vi "LoadCCDmode.vi"(8 "error in (no error)":errorcluster, 11 "S4GUI in":refnum<class "S4GUI.lvclass">) -> (0 "error out":errorcluster, 3 "S4GUI out":refnum<class "S4GUI.lvclass">)   [LabVIEW 2018, in "S4GUI.lvclass"]
uses:
  S4GUI.lvclass
  S4GUI.lvclass/S4GUI.ctl
  Acquisition/Acquisition.lvclass
  Interface/Interface.lvclass
  Channel/Channel.lvclass
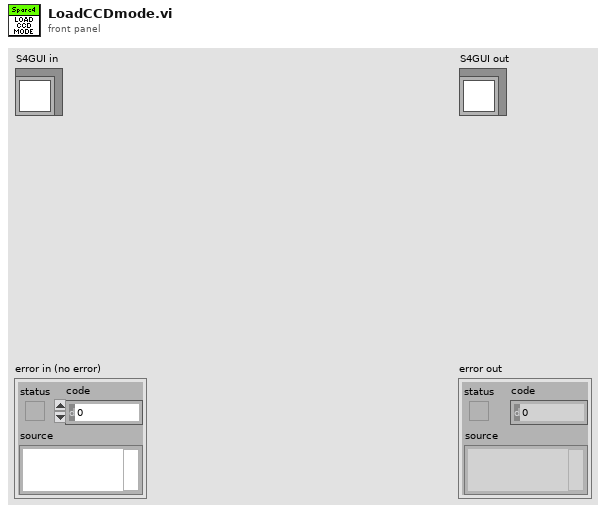
[diagram p1: front panel]
types:
  T1 = enum16{"SLOW BRIGHT: Conventional; 0.1 MHz; Gain 1", "SLOW FAINT: Conventional; 0.1 MHz; Gain 2", "NORMAL BRIGHT: Conventional; 1 MHz; Gain 1", "NORMAL FAINT: Conventional; 1 MHz; Gain 2", "FAST: EM; 10 MHz", "FAST+: EM; 20 MHz", "SUPERFAST: EM; 30 MHz"}
  T2 = enum16{"LARGE: FoV=5.6' / Pix=0.3\"", "LARGE: FoV=5.6' / Pix=0.7\"", "MEDIUM: FoV=2.8'/ Pix=0.3\"", "MEDIUM: FoV=2.8' / Pix=0.7\"", "SMALL FoV=1.4' / Pix=0.3\"", "SMALL: FoV=1.4' / Pix=0.7\""}
  T3 = cluster{"AcqRate":dbl, "MinExpTime":dbl, "readNoise":dbl, "readTime":dbl, "SatLim":dbl}
  T4 = cluster{"Image \nInitial Line":u16, "Image\nInitial Column":u16, "Image\nFinal Line":u16, "Image\nFInal Column":u16, "Vertical\nBinning":u16, "Horizontal\nBinning":u16, "Pre-amplification\nGain":u8, "CCD\nEM Gain":u16, "Readout\nRate":u8, "Shutter\nOpenning Time":i32, "Shutter\nClosing Time":i32, "Vertical\nShift Speed":u8, "Read\nMode":u8, "Vertical\nClock Voltage":u8, "A/D \nChannel":u32, "Shutter\nMode":u16, "Shutter\nTTL":u16, "Trigger\nMode":u16, "Frame\nTransfer":bool, "Acquisition\nMode":u8, "CCD \nEM Mode":u8}
  T5 = cluster{"ACQUISITION_MODE":u8, "TRIGGER_MODE":u8, "READ_MODE":u8, "PREAMP":u8, "READOUT_RATE":u8, "VERTICAL_SHIFT_SPEED":u8, "EM_MODE":u8, "EM_GAIN":u16, "SHUTTER_MODE":u8, "SHUTTER_TTL":u8, "SHUTTER_OPENING_TIME":u16, "SHUTTER_CLOSING_TIME":u16, "VBIN":u16, "HBIN":u16, "INITIAL_LINE":u16, "INITIAL_COLUMN":u16, "FINAL_LINE":u16, "FINAL_COLUMN":u16, "FRAME_TRANSFER":bool, "VERTICAL_CLOCK_VOLTAGE":u8, "AD_CHANNEL":u32}
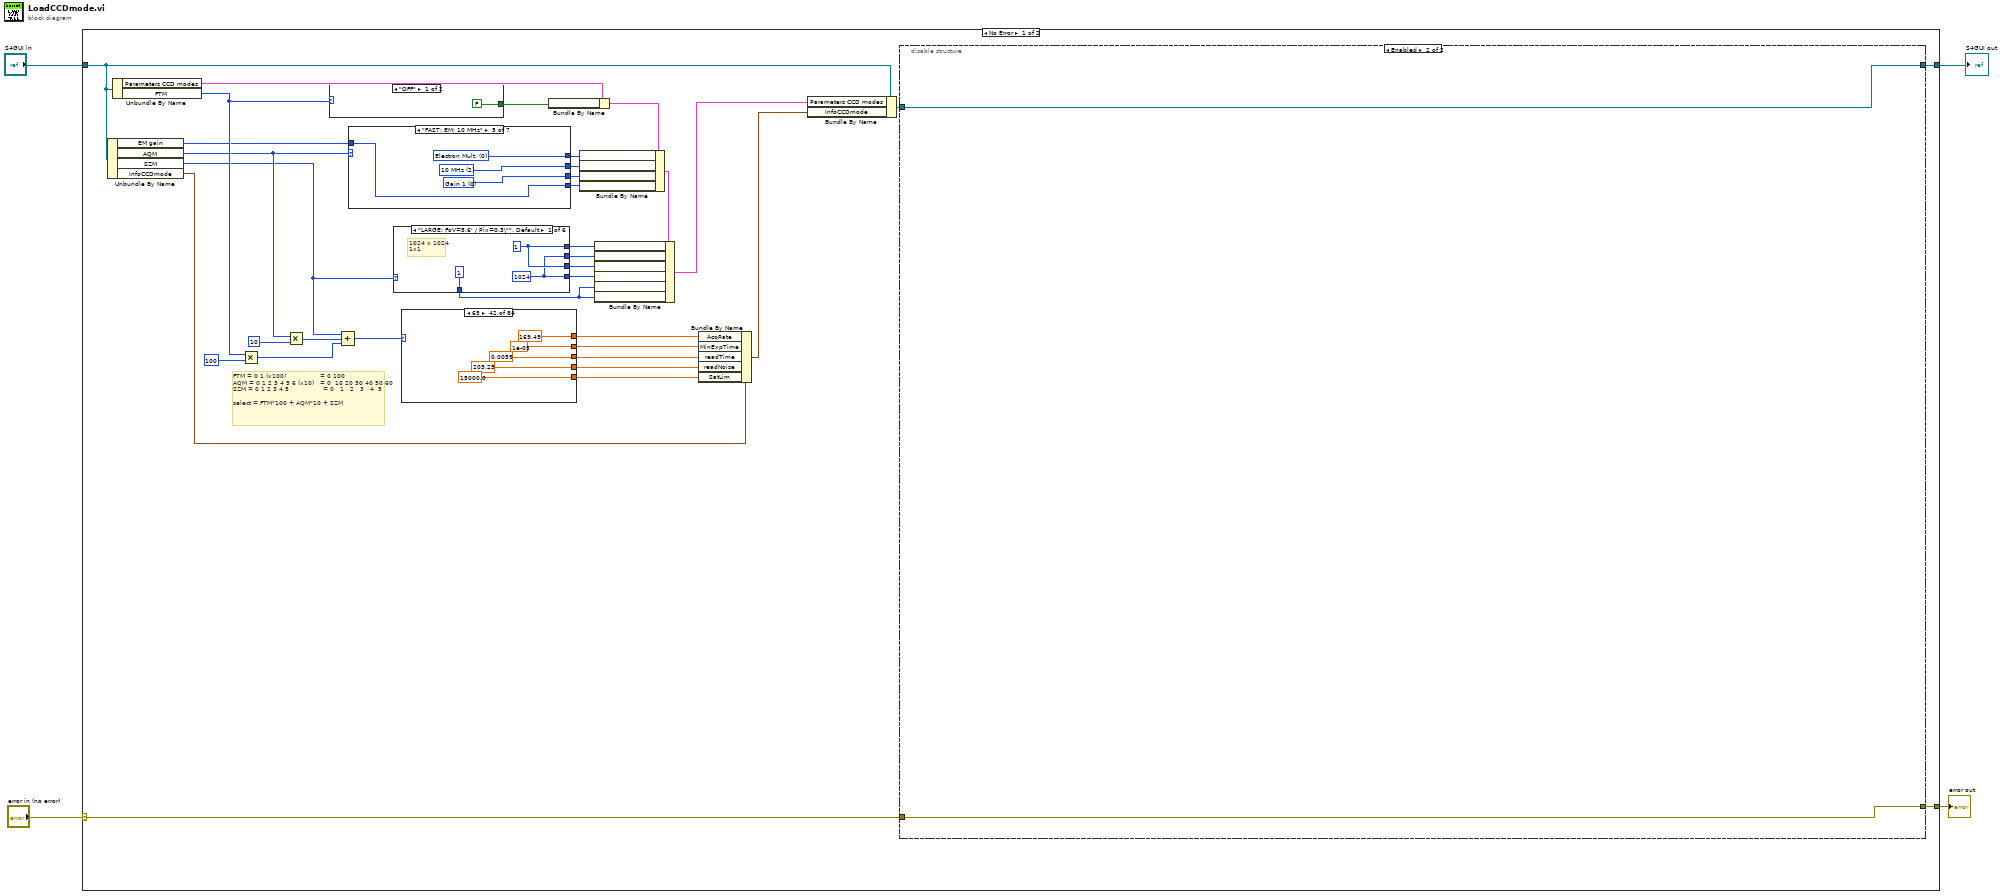
[diagram p0: block diagram]
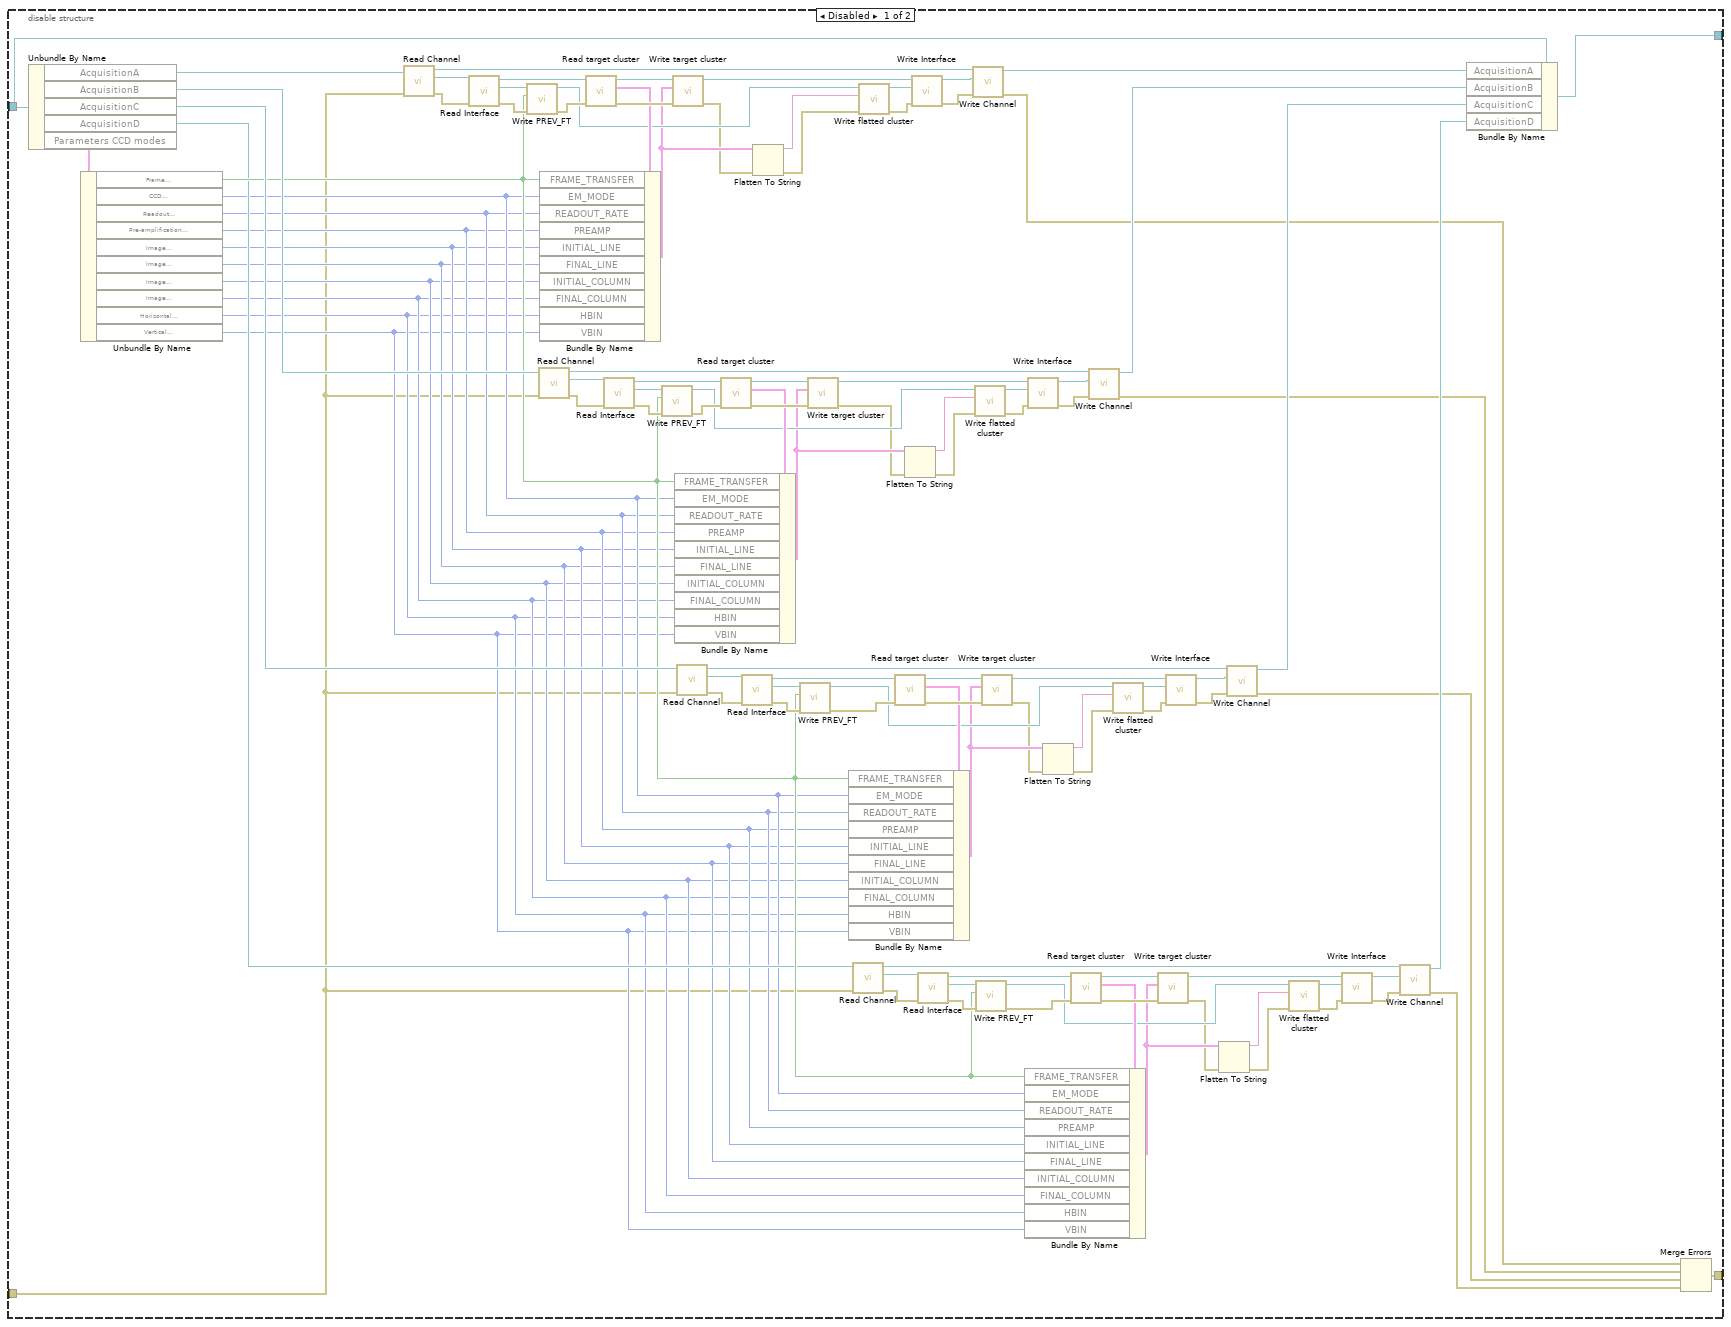
[diagram p2: hidden frame]
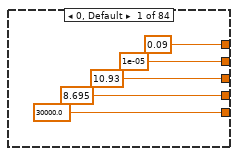
[diagram p3: hidden frame]
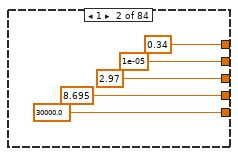
[diagram p4: hidden frame]
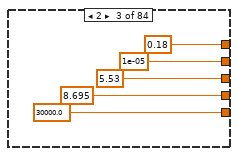
[diagram p5: hidden frame]
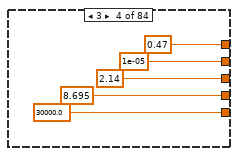
[diagram p6: hidden frame]
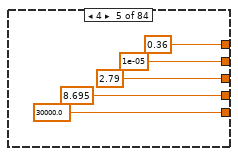
[diagram p7: hidden frame]
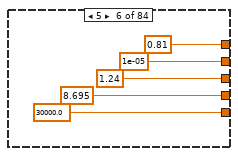
[diagram p8: hidden frame]
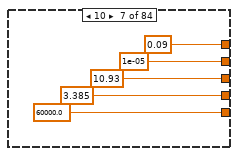
[diagram p9: hidden frame]
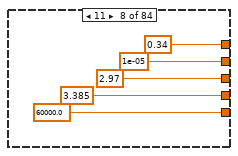
[diagram p10: hidden frame]
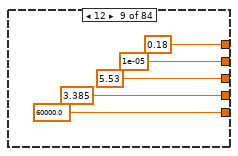
[diagram p11: hidden frame]
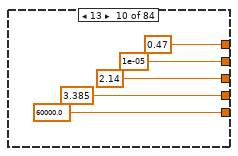
[diagram p12: hidden frame]
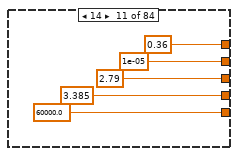
[diagram p13: hidden frame]
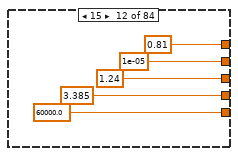
[diagram p14: hidden frame]
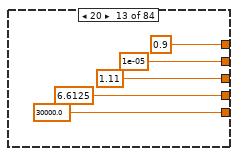
[diagram p15: hidden frame]
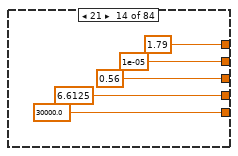
[diagram p16: hidden frame]
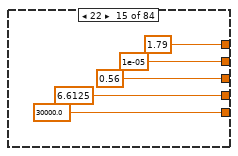
[diagram p17: hidden frame]
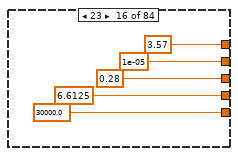
[diagram p18: hidden frame]
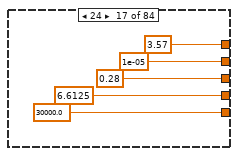
[diagram p19: hidden frame]
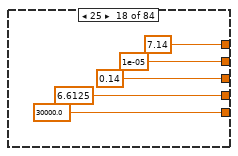
[diagram p20: hidden frame]
diagram:
  n1 = case shown="No Error" "error in (no error)" {
    selector: "error in (no error)" -> [w25 w618]
    tunnel: [w24 w618] -> w3
    tunnel: [w27 w617] -> w1
    tunnel: "S4GUI in" -> [w26 w617]
    frame No Error {
      # "FTM = 0 1 (x100)                 = 0 100\nAQM = 0 1 2 3 4 5 6 (x10)   = 0  10 20 30 40 50 60\nSZM = 0 1 2 3 4 5                 = 0   1   2   3   4  5\n\nselect = FTM*100 + AQM*10 + SZM"
      n2 = Unbundle By Name(w26) -> ("EM gain"=w5:u16, "AQM"=w8:T1, "SZM"=w7:T2, "InfoCCDmode"=w22:T3)
      n3 = Unbundle By Name(w26) -> ("Parameters CCD modes"=w20:T4, "FTM"=w9:enum16{"OFF", "ON"})
      n4 = Multiply(x=w9, y=100) -> (x*y=w11:i32)
      n5 = Multiply(x=w8, y=10) -> (x*y=w14:i32)
      n6 = case shown="\"OFF\"" w9 {
        tunnel: [FALSE TRUE] -> w39
        frame "OFF" {
        }
        frame "ON", Default {
        }
      }
      n7 = Compound Arithmetic op=ADD(w7, w14, w11) -> (w10:i32)
      n8 = case shown="\"FAST: EM; 10 MHz\"" w8 {
        tunnel: [w590 w594 w598 w602 w606 w610 w614] -> w37
        tunnel: [w589 w593 w597 w601 w604 w608 w612] -> w36
        tunnel: [w588 w592 w596 w600 w605 w609 w613] -> w35
        tunnel: [u16 2 u16 2 u16 2 u16 2 w603 w607 w611] -> w6
        tunnel: w5 -> [_ _ _ _ w603 w607 w611]
        frame "SLOW BRIGHT: Conventional; 0.1 MHz; Gain 1" {
          w588 = u8 0 items=["Gain 1", "Gain 2"] ("Pre-amplification\nGain")
          w589 = u8 1 items=["1 MHz", "0.1 MHz"] ("Readout\nRate")
          w590 = u8 1 items=["Electron Mult.", "Conventional"] ("CCD \nEM Mode")
        }
        frame "SLOW FAINT: Conventional; 0.1 MHz; Gain 2" {
          w592 = u8 1 items=["Gain 1", "Gain 2"] ("Pre-amplification\nGain")
          w593 = u8 1 items=["1 MHz", "0.1 MHz"] ("Readout\nRate")
          w594 = u8 1 items=["Electron Mult.", "Conventional"] ("CCD \nEM Mode")
        }
        frame "NORMAL BRIGHT: Conventional; 1 MHz; Gain 1", Default {
          w596 = u8 0 items=["Gain 1", "Gain 2"] ("Pre-amplification\nGain")
          w597 = u8 0 items=["1 MHz", "0.1 MHz"] ("Readout\nRate")
          w598 = u8 1 items=["Electron Mult.", "Conventional"] ("CCD \nEM Mode")
        }
        frame "NORMAL FAINT: Conventional; 1 MHz; Gain 2" {
          w600 = u8 1 items=["Gain 1", "Gain 2"] ("Pre-amplification\nGain")
          w601 = u8 0 items=["1 MHz", "0.1 MHz"] ("Readout\nRate")
          w602 = u8 1 items=["Electron Mult.", "Conventional"] ("CCD \nEM Mode")
        }
        frame "FAST: EM; 10 MHz" {
          w604 = u8 2 items=["30 MHz", "20 MHz", "10 MHz"] ("Readout\nRate")
          w605 = u8 0 items=["Gain 1", "Gain 2"] ("Pre-amplification\nGain")
          w606 = u8 0 items=["Electron Mult.", "Conventional"] ("CCD \nEM Mode")
        }
        frame "FAST+: EM; 20 MHz" {
          w608 = u8 1 items=["30 MHz", "20 MHz", "10 MHz"] ("Readout\nRate")
          w609 = u8 0 items=["Gain 1", "Gain 2"] ("Pre-amplification\nGain")
          w610 = u8 0 items=["Electron Mult.", "Conventional"] ("CCD \nEM Mode")
        }
        frame "SUPERFAST: EM; 30 MHz" {
          w612 = u8 0 items=["30 MHz", "20 MHz", "10 MHz"] ("Readout\nRate")
          w613 = u8 0 items=["Gain 1", "Gain 2"] ("Pre-amplification\nGain")
          w614 = u8 0 items=["Electron Mult.", "Conventional"] ("CCD \nEM Mode")
        }
      }
      n9 = case shown="\"LARGE: FoV=5.6' / Pix=0.3\\\"\", Default" w7 {
        tunnel: [w571 w574 w577 w579 w583 w585] -> w32
        tunnel: [w571 w574 w577 w579 w583 w585] -> w31
        tunnel: [w570 w573 w576 w580 w582 w586] -> w30
        tunnel: [w570 w573 w576 w580 w582 w586] -> w29
        tunnel: [1 2 1 2 1 2] -> w23
        frame "LARGE: FoV=5.6' / Pix=0.3\"", Default {
          w570 = 1024
          w571 = 1
          # "1024 x 1024\n1x1"
        }
        frame "LARGE: FoV=5.6' / Pix=0.7\"" {
          w573 = 1024
          w574 = 1
          # "1024x1024\n2x2"
        }
        frame "MEDIUM: FoV=2.8'/ Pix=0.3\"" {
          w576 = 768
          w577 = 257
          # "512x512\n1x1"
        }
        frame "MEDIUM: FoV=2.8' / Pix=0.7\"" {
          w580 = 768
          w579 = 257
          # "512x512\n1x1"
        }
        frame "SMALL FoV=1.4' / Pix=0.3\"" {
          w582 = 640
          w583 = 385
          # "256 x 256\n1x1"
        }
        frame "SMALL: FoV=1.4' / Pix=0.7\"" {
          w586 = 640
          w585 = 385
          # "256 x 256\n2x2"
        }
      }
      n10 = case shown="65" w10 {
        tunnel: [0.09 ("AcqRate") 0.34 ("AcqRate") 0.18 ("AcqRate") 0.47 ("AcqRate") 0.36 ("AcqRate") 0.81 ("AcqRate") 0.09 ("AcqRate") 0.34 ("AcqRate") 0.18 ("AcqRate") 0.47 ("AcqRate") 0.36 ("AcqRate") 0.81 ("AcqRate") 0.9 ("AcqRate") 1.79 ("AcqRate") 1.79 ("AcqRate") 3.57 ("AcqRate") 3.57 ("AcqRate") 7.14 ("AcqRate") 0.9 ("AcqRate") 1.79 ("AcqRate") 1.79 ("AcqRate") 3.57 ("AcqRate") 3.57 ("AcqRate") 7.14 ("AcqRate") 9.09 ("AcqRate") 17.54 ("AcqRate") 17.54 ("AcqRate") 34.48 ("AcqRate") 34.48 ("AcqRate") 66.67 ("AcqRate") 17.54 ("AcqRate") 34.48 ("AcqRate") 34.48 ("AcqRate") 66.67 ("AcqRate") 66.67 ("AcqRate") 120.48 ("AcqRate") 25.64 ("AcqRate") 50.0 ("AcqRate") 50.0 ("AcqRate") 90.91 ("AcqRate") 90.91 ("AcqRate") 169.49 ("AcqRate") 0.09 ("AcqRate") 0.34 ("AcqRate") 0.18 ("AcqRate") 0.47 ("AcqRate") 0.36 ("AcqRate") 0.81 ("AcqRate") 0.09 ("AcqRate") 0.34 ("AcqRate") 0.18 ("AcqRate") 0.47 ("AcqRate") 0.36 ("AcqRate") 0.81 ("AcqRate") 0.9 ("AcqRate") 1.79 ("AcqRate") 1.79 ("AcqRate") 3.57 ("AcqRate") 3.57 ("AcqRate") 7.14 ("AcqRate") 0.9 ("AcqRate") 1.79 ("AcqRate") 1.79 ("AcqRate") 3.57 ("AcqRate") 3.57 ("AcqRate") 7.14 ("AcqRate") 9.09 ("AcqRate") 17.54 ("AcqRate") 17.54 ("AcqRate") 34.48 ("AcqRate") 34.48 ("AcqRate") 66.67 ("AcqRate") 17.54 ("AcqRate") 34.48 ("AcqRate") 34.48 ("AcqRate") 66.67 ("AcqRate") 66.67 ("AcqRate") 120.48 ("AcqRate") 25.64 ("AcqRate") 50.0 ("AcqRate") 50.0 ("AcqRate") 90.91 ("AcqRate") 90.91 ("AcqRate") 169.49 ("AcqRate")] -> w19
        tunnel: [1e-05 ("AcqRate") 1e-05 ("AcqRate") 1e-05 ("AcqRate") 1e-05 ("AcqRate") 1e-05 ("AcqRate") 1e-05 ("AcqRate") 1e-05 ("AcqRate") 1e-05 ("AcqRate") 1e-05 ("AcqRate") 1e-05 ("AcqRate") 1e-05 ("AcqRate") 1e-05 ("AcqRate") 1e-05 ("AcqRate") 1e-05 ("AcqRate") 1e-05 ("AcqRate") 1e-05 ("AcqRate") 1e-05 ("AcqRate") 1e-05 ("AcqRate") 1e-05 ("AcqRate") 1e-05 ("AcqRate") 1e-05 ("AcqRate") 1e-05 ("AcqRate") 1e-05 ("AcqRate") 1e-05 ("AcqRate") 1e-05 ("AcqRate") 1e-05 ("AcqRate") 1e-05 ("AcqRate") 1e-05 ("AcqRate") 1e-05 ("AcqRate") 1e-05 ("AcqRate") 1e-05 ("AcqRate") 1e-05 ("AcqRate") 1e-05 ("AcqRate") 1e-05 ("AcqRate") 1e-05 ("AcqRate") 1e-05 ("AcqRate") 1e-05 ("AcqRate") 1e-05 ("AcqRate") 1e-05 ("AcqRate") 1e-05 ("AcqRate") 1e-05 ("AcqRate") 1e-05 ("AcqRate") 10.93 ("AcqRate") 2.97 ("AcqRate") 5.53 ("AcqRate") 2.14 ("AcqRate") 2.79 ("AcqRate") 1.24 ("AcqRate") 10.93 ("AcqRate") 2.97 ("AcqRate") 5.53 ("AcqRate") 2.14 ("AcqRate") 2.79 ("AcqRate") 1.24 ("AcqRate") 1.11 ("AcqRate") 0.56 ("AcqRate") 0.56 ("AcqRate") 0.28 ("AcqRate") 0.28 ("AcqRate") 0.14 ("AcqRate") 1.11 ("AcqRate") 0.56 ("AcqRate") 0.56 ("AcqRate") 0.28 ("AcqRate") 0.28 ("AcqRate") 0.14 ("AcqRate") 0.11 ("AcqRate") 0.057 ("AcqRate") 0.057 ("AcqRate") 0.029 ("AcqRate") 0.029 ("AcqRate") 0.015 ("AcqRate") 0.057 ("AcqRate") 0.029 ("AcqRate") 0.029 ("AcqRate") 0.015 ("AcqRate") 0.015 ("AcqRate") 0.0083 ("AcqRate") 0.039 ("AcqRate") 0.02 ("AcqRate") 0.02 ("AcqRate") 0.011 ("AcqRate") 0.011 ("AcqRate") 0.0059 ("AcqRate")] -> w18
        tunnel: [10.93 ("AcqRate") 2.97 ("AcqRate") 5.53 ("AcqRate") 2.14 ("AcqRate") 2.79 ("AcqRate") 1.24 ("AcqRate") 10.93 ("AcqRate") 2.97 ("AcqRate") 5.53 ("AcqRate") 2.14 ("AcqRate") 2.79 ("AcqRate") 1.24 ("AcqRate") 1.11 ("AcqRate") 0.56 ("AcqRate") 0.56 ("AcqRate") 0.28 ("AcqRate") 0.28 ("AcqRate") 0.14 ("AcqRate") 1.11 ("AcqRate") 0.56 ("AcqRate") 0.56 ("AcqRate") 0.28 ("AcqRate") 0.28 ("AcqRate") 0.14 ("AcqRate") 0.11 ("AcqRate") 0.057 ("AcqRate") 0.057 ("AcqRate") 0.029 ("AcqRate") 0.029 ("AcqRate") 0.015 ("AcqRate") 0.057 ("AcqRate") 0.029 ("AcqRate") 0.029 ("AcqRate") 0.015 ("AcqRate") 0.015 ("AcqRate") 0.0083 ("AcqRate") 0.039 ("AcqRate") 0.02 ("AcqRate") 0.02 ("AcqRate") 0.011 ("AcqRate") 0.011 ("AcqRate") 0.0059 ("AcqRate") 10.93 ("AcqRate") 2.97 ("AcqRate") 5.53 ("AcqRate") 2.14 ("AcqRate") 2.79 ("AcqRate") 1.24 ("AcqRate") 10.93 ("AcqRate") 2.97 ("AcqRate") 5.53 ("AcqRate") 2.14 ("AcqRate") 2.79 ("AcqRate") 1.24 ("AcqRate") 1.11 ("AcqRate") 0.56 ("AcqRate") 0.56 ("AcqRate") 0.28 ("AcqRate") 0.28 ("AcqRate") 0.14 ("AcqRate") 1.11 ("AcqRate") 0.56 ("AcqRate") 0.56 ("AcqRate") 0.28 ("AcqRate") 0.28 ("AcqRate") 0.14 ("AcqRate") 0.11 ("AcqRate") 0.057 ("AcqRate") 0.057 ("AcqRate") 0.029 ("AcqRate") 0.029 ("AcqRate") 0.015 ("AcqRate") 0.057 ("AcqRate") 0.029 ("AcqRate") 0.029 ("AcqRate") 0.015 ("AcqRate") 0.015 ("AcqRate") 0.083 ("AcqRate") 0.039 ("AcqRate") 0.02 ("AcqRate") 0.02 ("AcqRate") 0.011 ("AcqRate") 0.011 ("AcqRate") 0.0059 ("AcqRate")] -> w17
        tunnel: [8.695 ("AcqRate") 8.695 ("AcqRate") 8.695 ("AcqRate") 8.695 ("AcqRate") 8.695 ("AcqRate") 8.695 ("AcqRate") 3.385 ("AcqRate") 3.385 ("AcqRate") 3.385 ("AcqRate") 3.385 ("AcqRate") 3.385 ("AcqRate") 3.385 ("AcqRate") 6.6125 ("AcqRate") 6.6125 ("AcqRate") 6.6125 ("AcqRate") 6.6125 ("AcqRate") 6.6125 ("AcqRate") 6.6125 ("AcqRate") 4.7675 ("AcqRate") 4.7675 ("AcqRate") 4.7675 ("AcqRate") 4.7675 ("AcqRate") 4.7675 ("AcqRate") 4.7675 ("AcqRate") 78.05 ("AcqRate") 78.05 ("AcqRate") 78.05 ("AcqRate") 78.05 ("AcqRate") 78.05 ("AcqRate") 78.05 ("AcqRate") 146.25 ("AcqRate") 146.25 ("AcqRate") 146.25 ("AcqRate") 146.25 ("AcqRate") 146.25 ("AcqRate") 146.25 ("AcqRate") 203.25 ("AcqRate") 203.25 ("AcqRate") 203.25 ("AcqRate") 203.25 ("AcqRate") 203.25 ("AcqRate") 203.25 ("AcqRate") 8.695 ("AcqRate") 8.695 ("AcqRate") 8.695 ("AcqRate") 8.695 ("AcqRate") 8.695 ("AcqRate") 8.695 ("AcqRate") 3.385 ("AcqRate") 3.385 ("AcqRate") 3.385 ("AcqRate") 3.385 ("AcqRate") 3.385 ("AcqRate") 3.385 ("AcqRate") 6.6125 ("AcqRate") 6.6125 ("AcqRate") 6.6125 ("AcqRate") 6.6125 ("AcqRate") 6.6125 ("AcqRate") 6.6125 ("AcqRate") 4.7675 ("AcqRate") 4.7675 ("AcqRate") 4.7675 ("AcqRate") 4.7675 ("AcqRate") 4.7675 ("AcqRate") 4.7675 ("AcqRate") 78.05 ("AcqRate") 78.05 ("AcqRate") 78.05 ("AcqRate") 78.05 ("AcqRate") 78.05 ("AcqRate") 78.05 ("AcqRate") 146.25 ("AcqRate") 146.25 ("AcqRate") 146.25 ("AcqRate") 146.25 ("AcqRate") 146.25 ("AcqRate") 146.25 ("AcqRate") 203.25 ("AcqRate") 203.25 ("AcqRate") 203.25 ("AcqRate") 203.25 ("AcqRate") 203.25 ("AcqRate") 203.25 ("AcqRate")] -> w16
        tunnel: [30000.0 ("AcqRate") 30000.0 ("AcqRate") 30000.0 ("AcqRate") 30000.0 ("AcqRate") 30000.0 ("AcqRate") 30000.0 ("AcqRate") 60000.0 ("AcqRate") 60000.0 ("AcqRate") 60000.0 ("AcqRate") 60000.0 ("AcqRate") 60000.0 ("AcqRate") 60000.0 ("AcqRate") 30000.0 ("AcqRate") 30000.0 ("AcqRate") 30000.0 ("AcqRate") 30000.0 ("AcqRate") 30000.0 ("AcqRate") 30000.0 ("AcqRate") 60000.0 ("AcqRate") 60000.0 ("AcqRate") 60000.0 ("AcqRate") 60000.0 ("AcqRate") 60000.0 ("AcqRate") 60000.0 ("AcqRate") 15000.0 ("AcqRate") 15000.0 ("AcqRate") 15000.0 ("AcqRate") 15000.0 ("AcqRate") 15000.0 ("AcqRate") 15000.0 ("AcqRate") 15000.0 ("AcqRate") 15000.0 ("AcqRate") 15000.0 ("AcqRate") 15000.0 ("AcqRate") 15000.0 ("AcqRate") 15000.0 ("AcqRate") 15000.0 ("AcqRate") 15000.0 ("AcqRate") 15000.0 ("AcqRate") 15000.0 ("AcqRate") 15000.0 ("AcqRate") 15000.0 ("AcqRate") 30000.0 ("AcqRate") 30000.0 ("AcqRate") 30000.0 ("AcqRate") 30000.0 ("AcqRate") 30000.0 ("AcqRate") 30000.0 ("AcqRate") 60000.0 ("AcqRate") 60000.0 ("AcqRate") 60000.0 ("AcqRate") 60000.0 ("AcqRate") 60000.0 ("AcqRate") 60000.0 ("AcqRate") 30000.0 ("AcqRate") 30000.0 ("AcqRate") 30000.0 ("AcqRate") 30000.0 ("AcqRate") 30000.0 ("AcqRate") 30000.0 ("AcqRate") 60000.0 ("AcqRate") 60000.0 ("AcqRate") 60000.0 ("AcqRate") 60000.0 ("AcqRate") 60000.0 ("AcqRate") 60000.0 ("AcqRate") 15000.0 ("AcqRate") 15000.0 ("AcqRate") 15000.0 ("AcqRate") 15000.0 ("AcqRate") 15000.0 ("AcqRate") 15000.0 ("AcqRate") 15000.0 ("AcqRate") 15000.0 ("AcqRate") 15000.0 ("AcqRate") 15000.0 ("AcqRate") 15000.0 ("AcqRate") 15000.0 ("AcqRate") 15000.0 ("AcqRate") 15000.0 ("AcqRate") 15000.0 ("AcqRate") 15000.0 ("AcqRate") 15000.0 ("AcqRate") 15000.0 ("AcqRate")] -> w15
        frame 0, Default {
        }
        frame 1 {
        }
        frame 2 {
        }
        frame 3 {
        }
        frame 4 {
        }
        frame 5 {
        }
        frame 10 {
        }
        frame 11 {
        }
        frame 12 {
        }
        frame 13 {
        }
        frame 14 {
        }
        frame 15 {
        }
        frame 20 {
        }
        frame 21 {
        }
        frame 22 {
        }
        frame 23 {
        }
        frame 24 {
        }
        frame 25 {
        }
        frame 30 {
        }
        frame 31 {
        }
        frame 32 {
        }
        frame 33 {
        }
        frame 34 {
        }
        frame 35 {
        }
        frame 40 {
        }
        frame 41 {
        }
        frame 42 {
        }
        frame 43 {
        }
        frame 44 {
        }
        frame 45 {
        }
        frame 50 {
        }
        frame 51 {
        }
        frame 52 {
        }
        frame 53 {
        }
        frame 54 {
        }
        frame 55 {
        }
        frame 60 {
        }
        frame 61 {
        }
        frame 62 {
        }
        frame 63 {
        }
        frame 64 {
        }
        frame 65 {
        }
        frame 100 {
        }
        frame 101 {
        }
        frame 102 {
        }
        frame 103 {
        }
        frame 104 {
        }
        frame 105 {
        }
        frame 110 {
        }
        frame 111 {
        }
        frame 112 {
        }
        frame 113 {
        }
        frame 114 {
        }
        frame 115 {
        }
        frame 120 {
        }
        frame 121 {
        }
        frame 122 {
        }
        frame 123 {
        }
        frame 124 {
        }
        frame 125 {
        }
        frame 130 {
        }
        frame 131 {
        }
        frame 132 {
        }
        frame 133 {
        }
        frame 134 {
        }
        frame 135 {
        }
        frame 140 {
        }
        frame 141 {
        }
        frame 142 {
        }
        frame 143 {
        }
        frame 144 {
        }
        frame 145 {
        }
        frame 150 {
        }
        frame 151 {
        }
        frame 152 {
        }
        frame 153 {
        }
        frame 154 {
        }
        frame 155 {
        }
        frame 160 {
        }
        frame 161 {
        }
        frame 162 {
        }
        frame 163 {
        }
        frame 164 {
        }
        frame 165 {
        }
      }
      n11 = Bundle By Name(cluster=w20, "Frame\nTransfer"=w39) -> (w38:T4)
      n12 = Bundle By Name(cluster=w38, "CCD \nEM Mode"=w37, "Readout\nRate"=w36, "Pre-amplification\nGain"=w35, "CCD\nEM Gain"=w6) -> (w34:T4)
      n13 = Bundle By Name(cluster=w34, "Image \nInitial Line"=w32, "Image\nFinal Line"=w29, "Image\nInitial Column"=w31, "Image\nFInal Column"=w30, "Horizontal\nBinning"=w23, "Vertical\nBinning"=w23) -> (w33:T4)
      n14 = Bundle By Name(cluster=w22, "AcqRate"=w19, "MinExpTime"=w18, "readTime"=w17, "readNoise"=w16, "SatLim"=w15) -> (w21:T3)
      n15 = Bundle By Name(cluster=w26, "Parameters CCD modes"=w33, "InfoCCDmode"=w21) -> (w28:refnum<class "S4GUI.lvclass">)
      n16 = disable-structure shown="Enabled" {
        disable-tunnel: w28 -> [w127 w148]
        disable-tunnel: [w126 w148] -> w27
        disable-tunnel: w25 -> [w45 w147]
        disable-tunnel: [w40 w147] -> w24
        frame Disabled {
          n17 = Unbundle By Name(w127) -> ("AcquisitionA"=w146:refnum<class "Acquisition.lvclass">, "AcquisitionB"=w103:refnum<class "Acquisition.lvclass">, "AcquisitionC"=w82:refnum<class "Acquisition.lvclass">, "AcquisitionD"=w61:refnum<class "Acquisition.lvclass">, "Parameters CCD modes"=w128:T4)
          n18 = Unbundle By Name(w128) -> ("Frame\nTransfer"=w62:bool, "CCD \nEM Mode"=w54:u8, "Readout\nRate"=w53:u8, "Pre-amplification\nGain"=w52:u8, "Image \nInitial Line"=w51:u16, "Image\nFinal Line"=w50:u16, "Image\nInitial Column"=w49:u16, "Image\nFInal Column"=w48:u16, "Horizontal\nBinning"=w47:u16, "Vertical\nBinning"=w46:u16)
          n19 = call-dynamic "Read Channel.vi"("error in (no error)"=w45, "Acquisition in"=w146) -> ("error out"=w55:errorcluster, "Channel.lvclass"=w130:refnum<class "Channel.lvclass">, "Acquisition out"=w125:refnum<class "Acquisition.lvclass">)  [unwired: 7 in]
          n20 = call-dynamic "Read Interface.vi"("error in (no error)"=w55, "Channel in"=w130) -> ("error out"=w142:errorcluster, "Interface.lvclass"=w143:refnum<class "Interface.lvclass">, "Channel out"=w137:refnum<class "Channel.lvclass">)  [unwired: 7 in]
          n21 = call-dynamic "Write PREV_FT.vi"("error in (no error)"=w142, "PREV_FT"=w62, "Interface in"=w143) -> ("error out"=w141:errorcluster, "Interface out"=w138:refnum<class "Interface.lvclass">)  [unwired: 7 in]
          n22 = call-dynamic "Read Channel.vi"("error in (no error)"=w45, "Acquisition in"=w103) -> ("error out"=w56:errorcluster, "Channel.lvclass"=w107:refnum<class "Channel.lvclass">, "Acquisition out"=w105:refnum<class "Acquisition.lvclass">)  [unwired: 7 in]
          n23 = call-dynamic "Read target cluster.vi"("error in (no error)"=w141, "Channel in"=w137) -> ("error out"=w140:errorcluster, "target cluster"=w139:T5, "Channel out"=w136:refnum<class "Channel.lvclass">)  [unwired: 7 in]
          n24 = Bundle By Name(cluster=w139, "FRAME_TRANSFER"=w62, "EM_MODE"=w54, "READOUT_RATE"=w53, "PREAMP"=w52, "INITIAL_LINE"=w51, "FINAL_LINE"=w50, "INITIAL_COLUMN"=w49, "FINAL_COLUMN"=w48, "HBIN"=w47, "VBIN"=w46) -> (w134:T5)
          n25 = call-dynamic "Read Interface.vi"("error in (no error)"=w56, "Channel in"=w107) -> ("error out"=w119:errorcluster, "Interface.lvclass"=w120:refnum<class "Interface.lvclass">, "Channel out"=w114:refnum<class "Channel.lvclass">)  [unwired: 7 in]
          n26 = call-dynamic "Write PREV_FT.vi"("error in (no error)"=w119, "PREV_FT"=w62, "Interface in"=w120) -> ("error out"=w118:errorcluster, "Interface out"=w115:refnum<class "Interface.lvclass">)  [unwired: 7 in]
          n27 = call-dynamic "Write target cluster.vi"("error in (no error)"=w140, "target cluster"=w134, "Channel in"=w136) -> ("error out"=w132:errorcluster, "Channel out"=w135:refnum<class "Channel.lvclass">)  [unwired: 7 in]
          n28 = call-dynamic "Read Channel.vi"("error in (no error)"=w45, "Acquisition in"=w82) -> ("error out"=w57:errorcluster, "Channel.lvclass"=w86:refnum<class "Channel.lvclass">, "Acquisition out"=w84:refnum<class "Acquisition.lvclass">)  [unwired: 7 in]
          n29 = call-dynamic "Read target cluster.vi"("error in (no error)"=w118, "Channel in"=w114) -> ("error out"=w117:errorcluster, "target cluster"=w116:T5, "Channel out"=w113:refnum<class "Channel.lvclass">)  [unwired: 7 in]
          n30 = Bundle By Name(cluster=w116, "FRAME_TRANSFER"=w62, "EM_MODE"=w54, "READOUT_RATE"=w53, "PREAMP"=w52, "INITIAL_LINE"=w51, "FINAL_LINE"=w50, "INITIAL_COLUMN"=w49, "FINAL_COLUMN"=w48, "HBIN"=w47, "VBIN"=w46) -> (w111:T5)
          n31 = call-dynamic "Read Interface.vi"("error in (no error)"=w57, "Channel in"=w86) -> ("error out"=w98:errorcluster, "Interface.lvclass"=w99:refnum<class "Interface.lvclass">, "Channel out"=w93:refnum<class "Channel.lvclass">)  [unwired: 7 in]
          n32 = Flatten To String(anything=w134, error in (no error)=w132) -> (data string=w133:string, error out=w131:errorcluster)  [unwired: 2 in, 1 out]
          n33 = call-dynamic "Write PREV_FT.vi"("error in (no error)"=w98, "PREV_FT"=w62, "Interface in"=w99) -> ("error out"=w97:errorcluster, "Interface out"=w94:refnum<class "Interface.lvclass">)  [unwired: 7 in]
          n34 = call-dynamic "Write target cluster.vi"("error in (no error)"=w117, "target cluster"=w111, "Channel in"=w113) -> ("error out"=w109:errorcluster, "Channel out"=w112:refnum<class "Channel.lvclass">)  [unwired: 7 in]
          n35 = call-dynamic "Read Channel.vi"("error in (no error)"=w45, "Acquisition in"=w61) -> ("error out"=w58:errorcluster, "Channel.lvclass"=w66:refnum<class "Channel.lvclass">, "Acquisition out"=w64:refnum<class "Acquisition.lvclass">)  [unwired: 7 in]
          n36 = call "Write flatted cluster.vi"("error in (no error)"=w131, "flatted cluster"=w133, "Interface in"=w138) -> ("error out"=w145:errorcluster, "Interface out"=w144:refnum<class "Interface.lvclass">)  [unwired: 7 in]
          n37 = call-dynamic "Read target cluster.vi"("error in (no error)"=w97, "Channel in"=w93) -> ("error out"=w96:errorcluster, "target cluster"=w95:T5, "Channel out"=w92:refnum<class "Channel.lvclass">)  [unwired: 7 in]
          n38 = Bundle By Name(cluster=w95, "FRAME_TRANSFER"=w62, "EM_MODE"=w54, "READOUT_RATE"=w53, "PREAMP"=w52, "INITIAL_LINE"=w51, "FINAL_LINE"=w50, "INITIAL_COLUMN"=w49, "FINAL_COLUMN"=w48, "HBIN"=w47, "VBIN"=w46) -> (w90:T5)
          n39 = Flatten To String(anything=w111, error in (no error)=w109) -> (data string=w110:string, error out=w108:errorcluster)  [unwired: 2 in, 1 out]
          n40 = call-dynamic "Write Interface.vi"("error in (no error)"=w145, "Interface.lvclass"=w144, "Channel in"=w135) -> ("error out"=w129:errorcluster, "Channel out"=w124:refnum<class "Channel.lvclass">)  [unwired: 7 in]
          n41 = call-dynamic "Read Interface.vi"("error in (no error)"=w58, "Channel in"=w66) -> ("error out"=w78:errorcluster, "Interface.lvclass"=w79:refnum<class "Interface.lvclass">, "Channel out"=w73:refnum<class "Channel.lvclass">)  [unwired: 7 in]
          n42 = call-dynamic "Write Channel.vi"("error in (no error)"=w129, "Channel.lvclass"=w124, "Acquisition in"=w125) -> ("error out"=w41:errorcluster, "Acquisition out"=w123:refnum<class "Acquisition.lvclass">)  [unwired: 7 in]
          n43 = call "Write flatted cluster.vi"("error in (no error)"=w108, "flatted cluster"=w110, "Interface in"=w115) -> ("error out"=w122:errorcluster, "Interface out"=w121:refnum<class "Interface.lvclass">)  [unwired: 7 in]
          n44 = call-dynamic "Write PREV_FT.vi"("error in (no error)"=w78, "PREV_FT"=w62, "Interface in"=w79) -> ("error out"=w77:errorcluster, "Interface out"=w74:refnum<class "Interface.lvclass">)  [unwired: 7 in]
          n45 = call-dynamic "Write target cluster.vi"("error in (no error)"=w96, "target cluster"=w90, "Channel in"=w92) -> ("error out"=w88:errorcluster, "Channel out"=w91:refnum<class "Channel.lvclass">)  [unwired: 7 in]
          n46 = call-dynamic "Write Interface.vi"("error in (no error)"=w122, "Interface.lvclass"=w121, "Channel in"=w112) -> ("error out"=w106:errorcluster, "Channel out"=w104:refnum<class "Channel.lvclass">)  [unwired: 7 in]
          n47 = Flatten To String(anything=w90, error in (no error)=w88) -> (data string=w89:string, error out=w87:errorcluster)  [unwired: 2 in, 1 out]
          n48 = call-dynamic "Read target cluster.vi"("error in (no error)"=w77, "Channel in"=w73) -> ("error out"=w76:errorcluster, "target cluster"=w75:T5, "Channel out"=w72:refnum<class "Channel.lvclass">)  [unwired: 7 in]
          n49 = Bundle By Name(cluster=w75, "FRAME_TRANSFER"=w62, "EM_MODE"=w54, "READOUT_RATE"=w53, "PREAMP"=w52, "INITIAL_LINE"=w51, "FINAL_LINE"=w50, "INITIAL_COLUMN"=w49, "FINAL_COLUMN"=w48, "HBIN"=w47, "VBIN"=w46) -> (w70:T5)
          n50 = call-dynamic "Write Channel.vi"("error in (no error)"=w106, "Channel.lvclass"=w104, "Acquisition in"=w105) -> ("error out"=w42:errorcluster, "Acquisition out"=w102:refnum<class "Acquisition.lvclass">)  [unwired: 7 in]
          n51 = call "Write flatted cluster.vi"("error in (no error)"=w87, "flatted cluster"=w89, "Interface in"=w94) -> ("error out"=w101:errorcluster, "Interface out"=w100:refnum<class "Interface.lvclass">)  [unwired: 7 in]
          n52 = call-dynamic "Write target cluster.vi"("error in (no error)"=w76, "target cluster"=w70, "Channel in"=w72) -> ("error out"=w68:errorcluster, "Channel out"=w71:refnum<class "Channel.lvclass">)  [unwired: 7 in]
          n53 = call-dynamic "Write Interface.vi"("error in (no error)"=w101, "Interface.lvclass"=w100, "Channel in"=w91) -> ("error out"=w85:errorcluster, "Channel out"=w83:refnum<class "Channel.lvclass">)  [unwired: 7 in]
          n54 = Flatten To String(anything=w70, error in (no error)=w68) -> (data string=w69:string, error out=w67:errorcluster)  [unwired: 2 in, 1 out]
          n55 = call-dynamic "Write Channel.vi"("error in (no error)"=w85, "Channel.lvclass"=w83, "Acquisition in"=w84) -> ("error out"=w43:errorcluster, "Acquisition out"=w60:refnum<class "Acquisition.lvclass">)  [unwired: 7 in]
          n56 = call "Write flatted cluster.vi"("error in (no error)"=w67, "flatted cluster"=w69, "Interface in"=w74) -> ("error out"=w81:errorcluster, "Interface out"=w80:refnum<class "Interface.lvclass">)  [unwired: 7 in]
          n57 = call-dynamic "Write Interface.vi"("error in (no error)"=w81, "Interface.lvclass"=w80, "Channel in"=w71) -> ("error out"=w65:errorcluster, "Channel out"=w63:refnum<class "Channel.lvclass">)  [unwired: 7 in]
          n58 = call-dynamic "Write Channel.vi"("error in (no error)"=w65, "Channel.lvclass"=w63, "Acquisition in"=w64) -> ("error out"=w44:errorcluster, "Acquisition out"=w59:refnum<class "Acquisition.lvclass">)  [unwired: 7 in]
          n59 = Bundle By Name(cluster=w127, "AcquisitionA"=w123, "AcquisitionB"=w102, "AcquisitionC"=w60, "AcquisitionD"=w59) -> (w126:refnum<class "S4GUI.lvclass">)
          n60 = Merge Errors(w41, w42, w43, w44) -> (w40:errorcluster)
        }
        frame Enabled {
        }
      }
    }
    frame Error {
    }
  }
  "error out" <- w3
  "S4GUI out" <- w1
